vi "Linear Space.vi"(4 "error in (no error)":errorcluster, 5 "Number of Samples":u32, 6 "Maximum":dbl, 7 "Minimum":dbl) -> (0 "error out":errorcluster, 3 "Array":dbl[](array[numeric]))   [LabVIEW 2014]
doc: "This subVI will create an evenly spaced array of elements equal to the Number of Samples between the Minimum and Maximum"
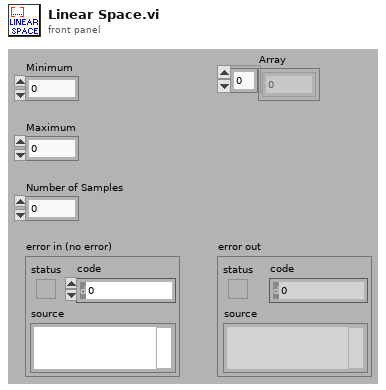
[diagram p1: front panel]
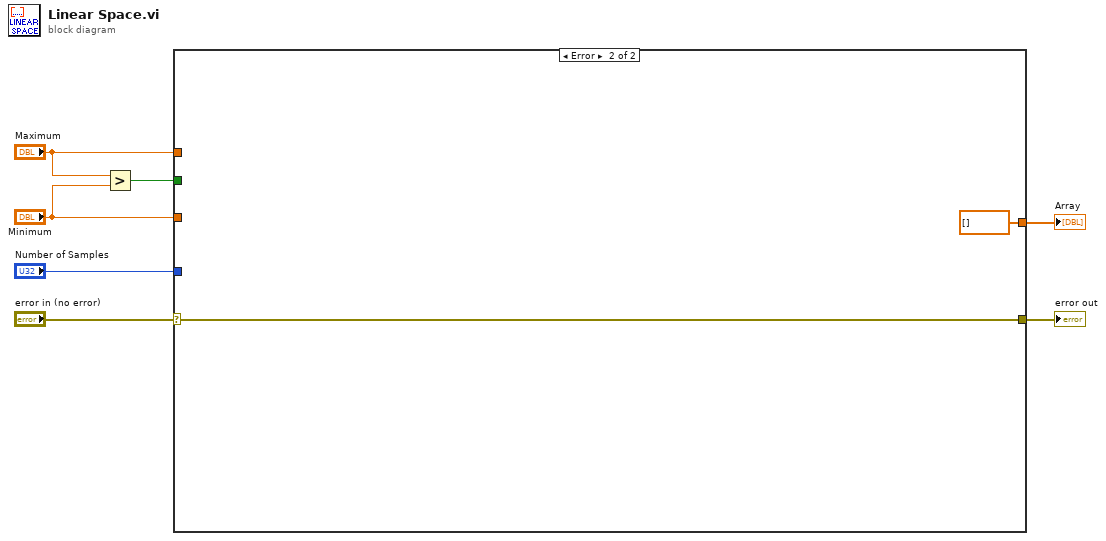
[diagram p0: block diagram]
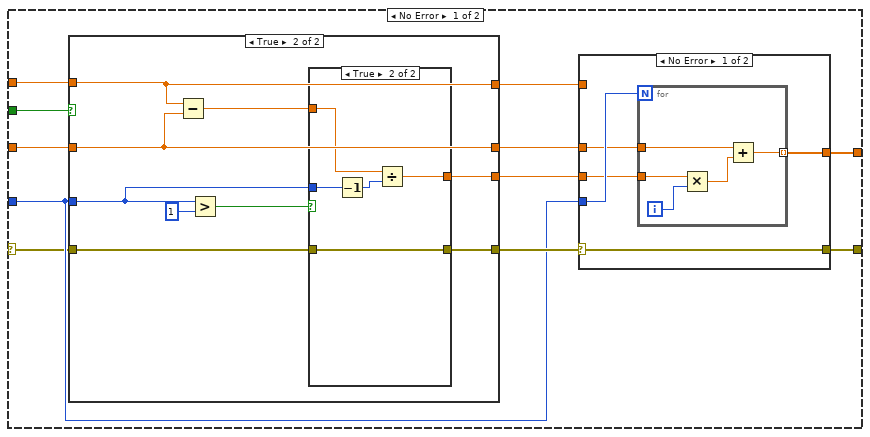
[diagram p2: hidden frame]
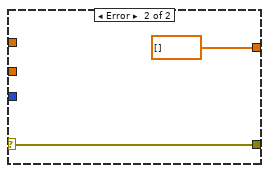
[diagram p3: hidden frame]
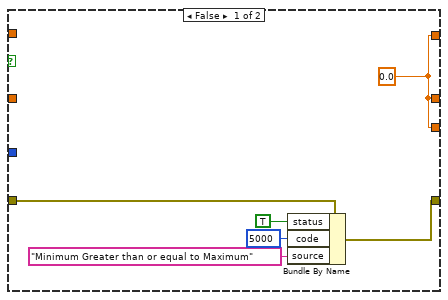
[diagram p4: hidden frame]
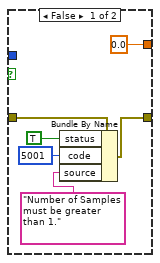
[diagram p5: hidden frame]
diagram:
  n1 = Greater?(x="Maximum", y="Minimum") -> (0:w7:bool)
  n2 = case shown="Error" "error in (no error)" {
    selector: "error in (no error)" -> [w8 w57]
    tunnel: w7 -> [w18 _]
    tunnel: "Maximum" -> [w17 _]
    tunnel: "Minimum" -> [w16 _]
    tunnel: [w14 w57] -> w4
    tunnel: "Number of Samples" -> [w10 _]
    tunnel: [w9 dbl[] []] -> w2
    frame No Error {
      n3 = case shown="True" w18 {
        tunnel: w8 -> [w36 w43]
        tunnel: [w32 w42] -> w15
        tunnel: w17 -> [_ w41]
        tunnel: w16 -> [_ w40]
        tunnel: w10 -> [_ w37]
        tunnel: [w31 w44] -> w13
        tunnel: [w31 w41] -> w12
        tunnel: [w31 w40] -> w11
        frame False {
          w31 = 0.0
          n4 = Bundle By Name(cluster=w36, "status"=TRUE, "code"=5000, "source"="Minimum Greater than or equal to Maximum") -> (w32:errorcluster)
        }
        frame True {
          n5 = Subtract(x=w41, y=w40) -> (x-y=w45:dbl)
          n6 = Greater?(x=w37, y=u32 1) -> (0:w38:bool)
          n7 = case shown="True" w38 {
            tunnel: w45 -> [_ w56]
            tunnel: [0.0 w55] -> w44
            tunnel: w43 -> [w50 w54]
            tunnel: [w49 w54] -> w42
            tunnel: w37 -> [_ w52]
            frame False {
              n8 = Bundle By Name(cluster=w50, "status"=TRUE, "code"=5001, "source"="Number of Samples must be greater than 1.") -> (w49:errorcluster)
            }
            frame True {
              n9 = Decrement(x=w52) -> (x-1=w53:u32)
              n10 = Divide(x=w56, y=w53) -> (x/y=w55:dbl)
            }
          }
        }
      }
      n11 = case shown="No Error" w15 {
        selector: w15 -> [w23 w29]
        tunnel: [w23 w29] -> w14
        tunnel: w13 -> [w20 _]
        tunnel: w12 -> [_ _]
        tunnel: w11 -> [w21 _]
        tunnel: w10 -> [w22 _]
        tunnel: [w19 dbl[] []] -> w9
        frame No Error {
          n12 = for {
            N: w22 -> [_]
            tunnel: w21 -> [w25]
            tunnel: w20 -> [w27]
            tunnel: [w24] -> w19 mode=indexing
            i -> [w28]
            n13 = Multiply(x=w27, y=w28) -> (x*y=w26:dbl)
            n14 = Add(x=w25, y=w26) -> (x+y=w24:dbl)
          }
        }
        frame Error {
        }
      }
    }
    frame Error {
    }
  }
  "error out" <- w4
  "Array" <- w2
